vi "init_constV.vi"() -> (1 "output_constV_parameters":T1)   [LabVIEW 2014, in "technique_parameters.lvclass"]
uses:
  technique_parameters.lvclass
panel:
  in  "Sense Range":T2(ring)
  in  "Sample Rate":dbl=100.0 min=0.01 max=100.0
  in  "Exert Time":i32 min=-1 max=360000000
  in  "Voltage Level":dbl min=-10.0 max=10.0
  in  "Exit":bool
  in  "Set":bool
  # "V"
  # "s / point"
  # "ms"
  # "A"
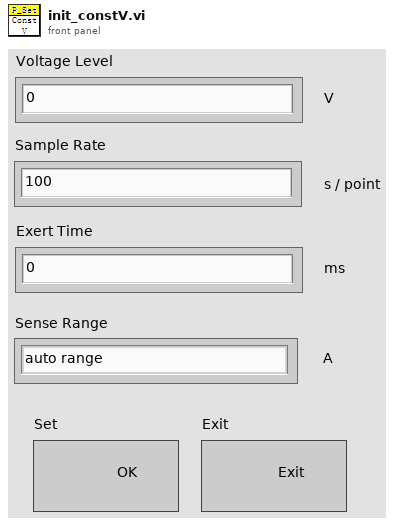
[diagram p1: front panel]
types:
  T1 = cluster{"volt_level/V":dbl, "exert_time/ms":u32, "sample_rate/(s/pt)":dbl, "sense_range/amp":enum16{"auto range", "1E-1", "1E-2", "1E-3", "1E-4", "1E-5", "1E-6", "1E-7", "1E-8", "1E-9"}}
  T2 = enum16{"auto range", "1E-1", "1E-2", "1E-3", "1E-4", "1E-5", "1E-6", "1E-7", "1E-8", "1E-9"}
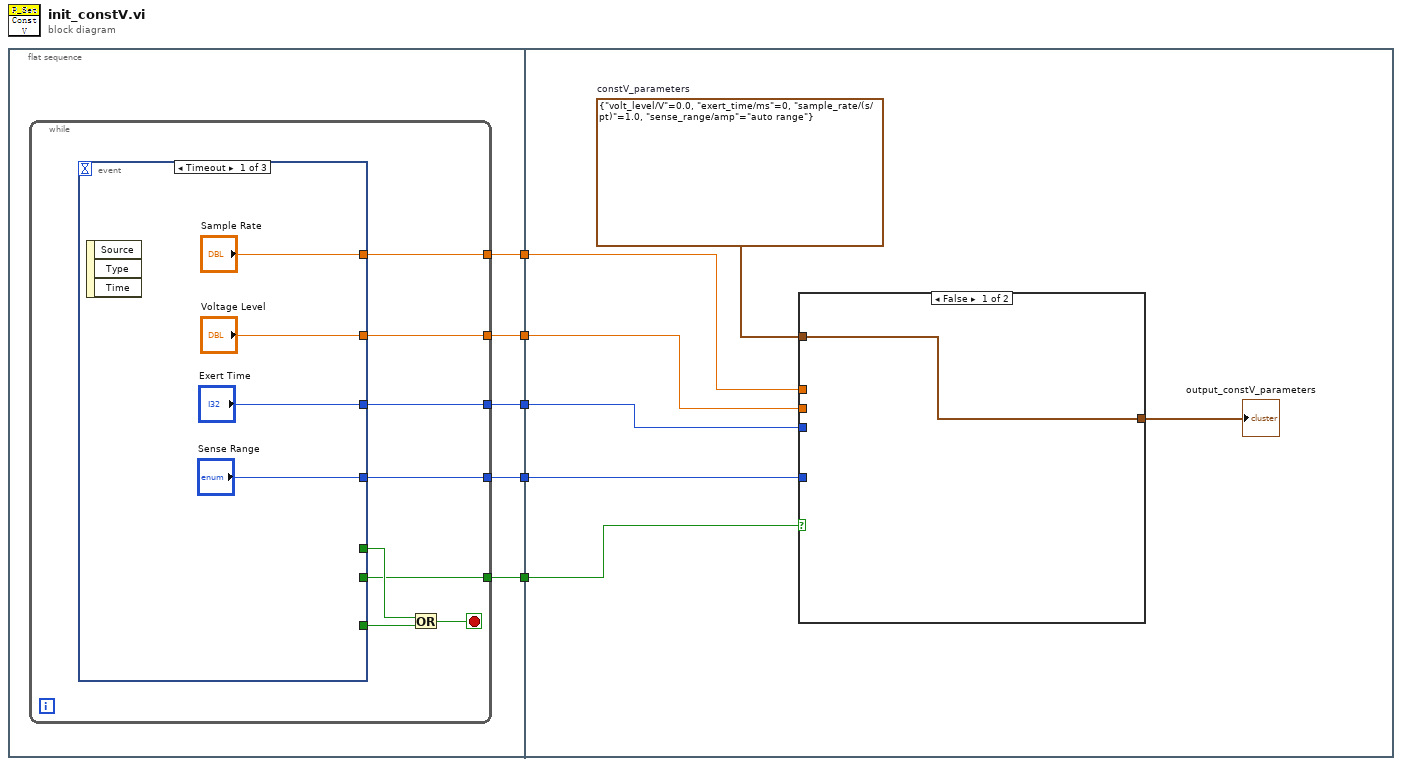
[diagram p0: block diagram]
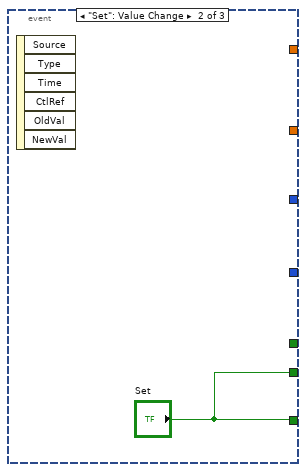
[diagram p2: hidden frame]
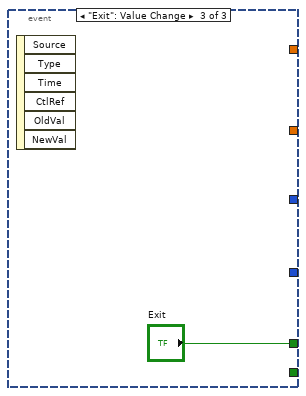
[diagram p3: hidden frame]
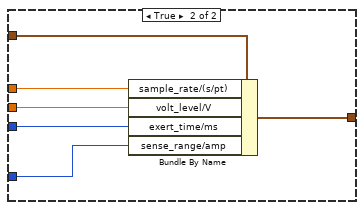
[diagram p4: hidden frame]
diagram:
  n1 = flat-sequence {
    tunnel: [w10] -> w5
    tunnel: [w9] -> w4
    tunnel: [w8] -> w3
    tunnel: [w7] -> w2
    tunnel: [w6] -> w1
    tunnel: w5 -> [w29]
    tunnel: w4 -> [w30]
    tunnel: w3 -> [w28]
    tunnel: w2 -> [w27]
    tunnel: w1 -> [w26]
    frame #0 {
      n2 = while {
        tunnel: [w18] -> w9
        tunnel: [w17] -> w10
        tunnel: [w16] -> w8
        tunnel: [w15] -> w7
        tunnel: [w11] -> w6
        stop <- w12 stop-if-true
        n3 = event shown="[0] Timeout" {
          selector: _ -> [_ _ _]
          dyn-events: _ -> [_ _ _]
          timeout: _ -> [_ _ _]
          tunnel: ["Sample Rate" _ _] -> w18
          tunnel: ["Voltage Level" _ _] -> w17
          tunnel: ["Exert Time" _ _] -> w16
          tunnel: ["Sense Range" _ _] -> w15
          tunnel: [_ _ "Exit"] -> w14
          tunnel: [_ "Set" _] -> w13
          tunnel: [_ "Set" _] -> w11
          event Timeout {
            n4 = event-data() -> ()  [unwired: 1 in, 3 out]
          }
          event "Set": Value Change {
            n5 = event-data() -> ()  [unwired: 1 in, 6 out]
          }
          event "Exit": Value Change {
            n6 = event-data() -> ()  [unwired: 1 in, 6 out]
          }
        }
        n7 = Or(x=w14, y=w13) -> (x .or. y?=w12:bool)
      }
    }
    frame #1 {
      w31 = T1 {"volt_level/V"=0.0, "exert_time/ms"=0, "sample_rate/(s/pt)"=1.0, "sense_range/amp"=enum."auto range"}  # constV_parameters
      n8 = case shown="False" w26 {
        tunnel: w31 -> [w32 w38]
        tunnel: w30 -> [_ w37]
        tunnel: w29 -> [_ w36]
        tunnel: w28 -> [_ w35]
        tunnel: w27 -> [_ w34]
        tunnel: [w32 w33] -> w25
        frame False {
        }
        frame True {
          n9 = Bundle By Name(cluster=w38, "sample_rate/(s/pt)"=w37, "volt_level/V"=w36, "exert_time/ms"=w35, "sense_range/amp"=w34) -> (w33:T1)
        }
      }
      "output_constV_parameters" <- w25
    }
  }
